vi "JKISM+ EventJKISM Module Example.vi"() -> ()   [LabVIEW 2014]
uses:
  user.lib/_NEVSTOP/JKI State Machine ++/JKI-State-Machine-Plus.lvlib
panel:
  in  "DoSth: DoC(error)":bool
  in  "DoSth: DoB":bool
  in  "DoSth: DoA":bool
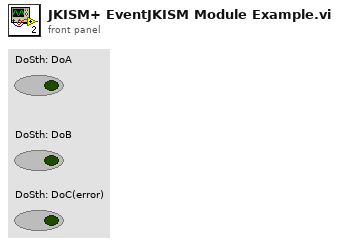
[diagram p1: front panel]
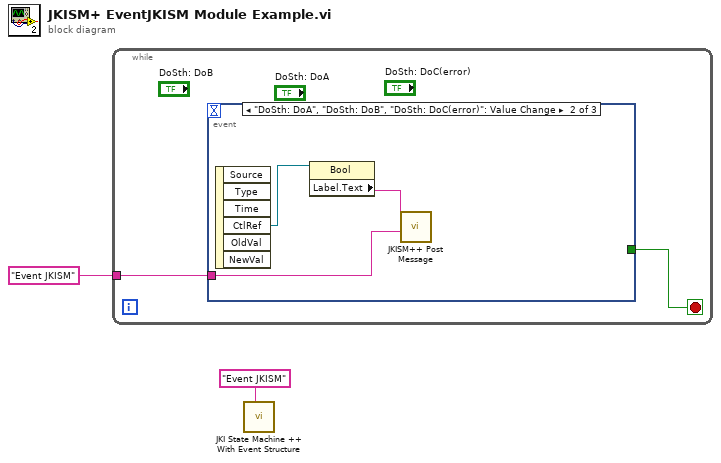
[diagram p0: block diagram]
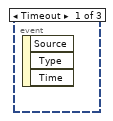
[diagram p2: hidden frame]
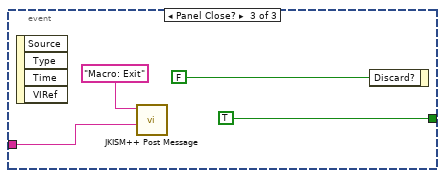
[diagram p3: hidden frame]
diagram:
  n1 = while {
    tunnel: "Event JKISM" ("Name(\"\" to use uuid)") -> [w3]
    stop <- w4 stop-if-true
    n2 = event shown="[1] \"DoSth: DoA\", \"DoSth: DoB\", \"DoSth: DoC(error)\": Value Change" {
      selector: _ -> [_ _ _]
      dyn-events: _ -> [_ _ _]
      timeout: _ -> [_ _ _]
      tunnel: [_ _ TRUE ("Discard?")] -> w4
      tunnel: w3 -> [_ w7 w8]
      event Timeout {
        n3 = event-data() -> ()  [unwired: 1 in, 3 out]
      }
      event "DoSth: DoA", "DoSth: DoB", "DoSth: DoC(error)": Value Change {
        n4 = event-data() -> ("CtlRef"=w6:refnum<vi>)  [unwired: 1 in, 5 out]
        n5 = property class="Bool"(reference=w6) -> ("Label.Text"=w5:string)  [unwired: 1 in, 2 out]
        n6 = call "JKISM++ Post Message.vi"("Dest Module"=w7, "States"=w5) -> ()  [unwired: 9 in, 1 out]
      }
      event Panel Close? {
        n7 = event-data() -> ()  [unwired: 1 in, 4 out]
        n8 = call "JKISM++ Post Message.vi"("Dest Module"=w8, "States"="Macro: Exit") -> ()  [unwired: 9 in, 1 out]
        n9 = event-data("Discard?"=FALSE) -> ()  [unwired: 1 in, 1 out]
      }
    }
  }
  n10 = call "JKI State Machine ++ With Event Structure.vi"("Name(\"\" to use uuid)"="Event JKISM" ("Name(\"\" to use uuid)")) -> ()  [unwired: 11 in]
